vi "质控单元流程.vi"   [LabVIEW 2016]
types:
  T1 = enum16{"步骤1", "步骤2", "步骤3", "步骤4", "步骤5", "步骤6", "步骤7", "步骤8", "步骤9", "步骤10"}
  T2 = enum32{"Bad", "Idle", "Run top level", "Running"}
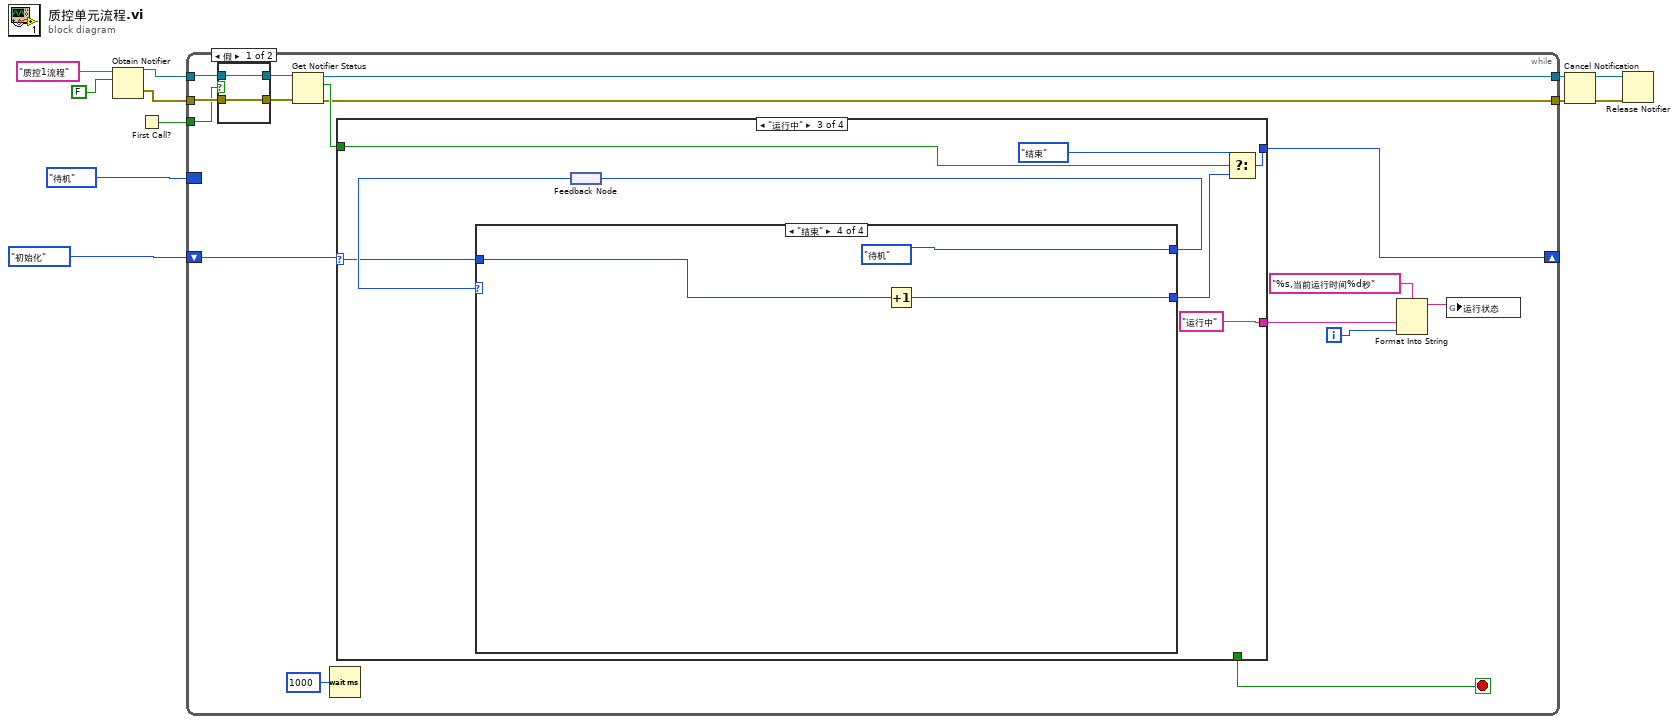
[diagram p0: block diagram]
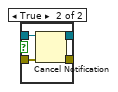
[diagram p2: hidden frame]
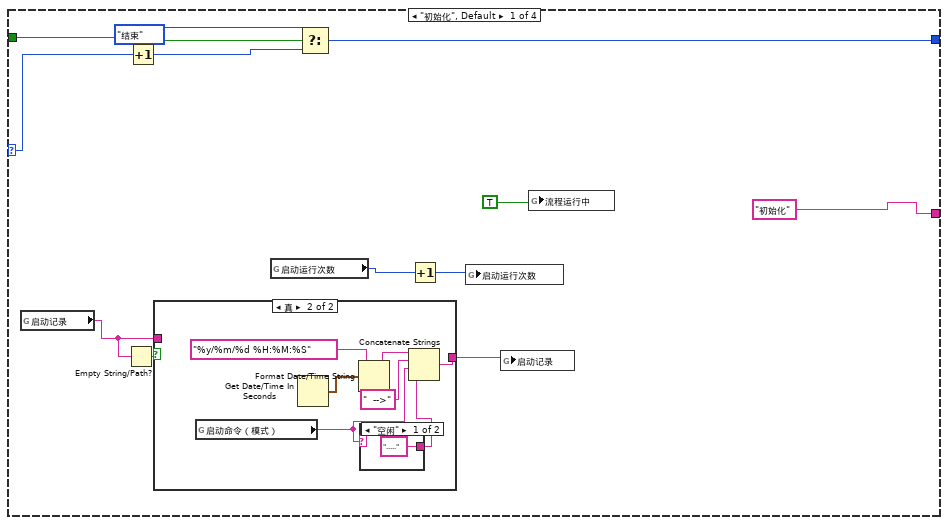
[diagram p3: hidden frame]
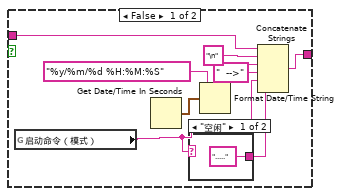
[diagram p4: hidden frame]
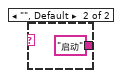
[diagram p5: hidden frame]
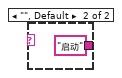
[diagram p6: hidden frame]
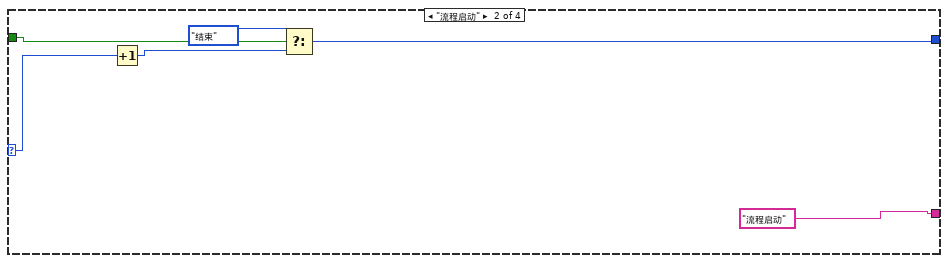
[diagram p7: hidden frame]
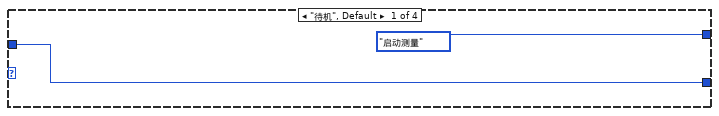
[diagram p8: hidden frame]
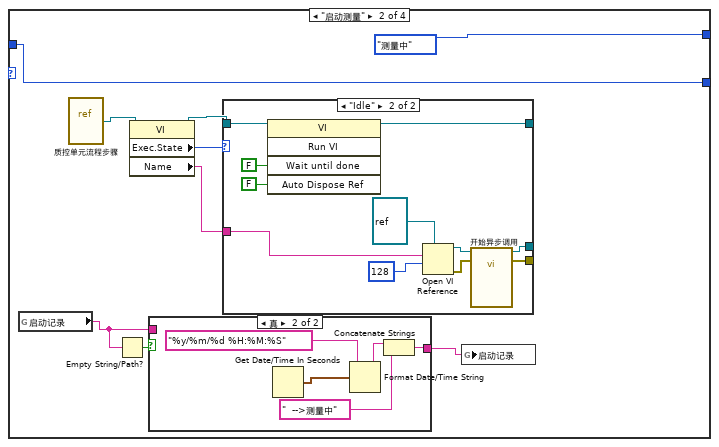
[diagram p9: hidden frame]
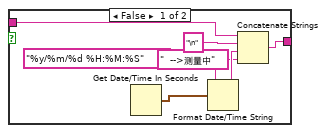
[diagram p10: hidden frame]
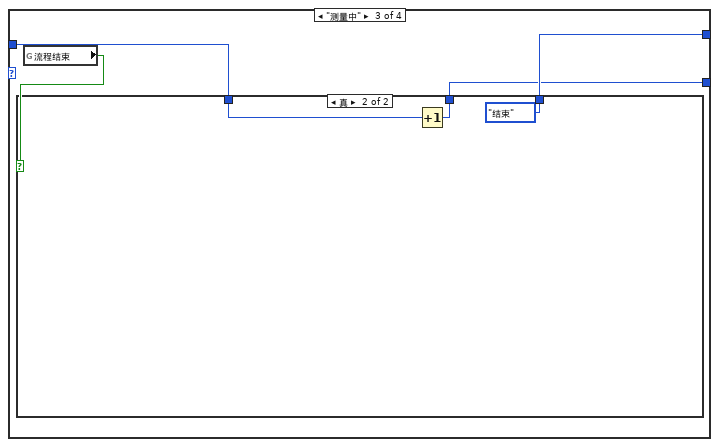
[diagram p12: hidden frame]
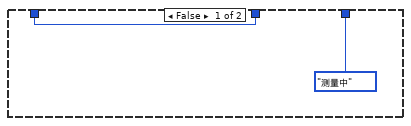
[diagram p13: hidden frame]
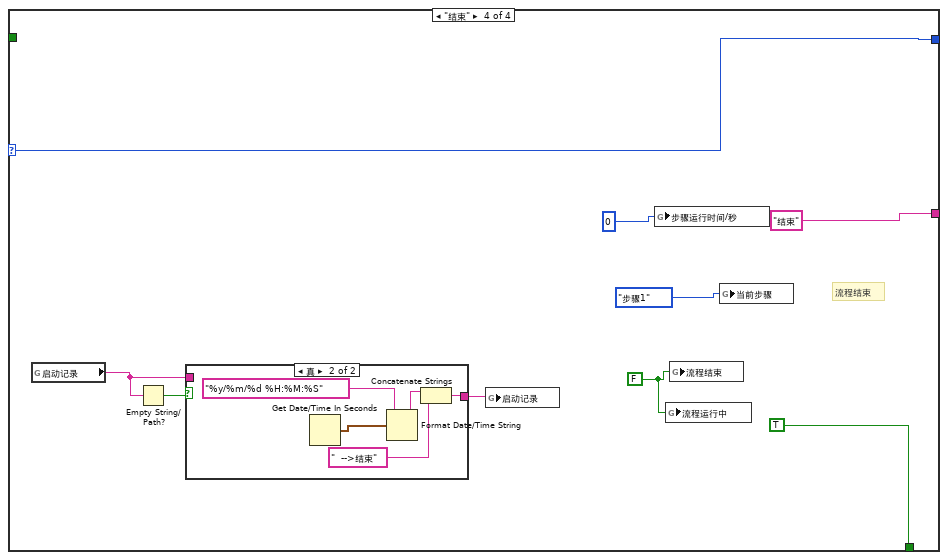
[diagram p14: hidden frame]
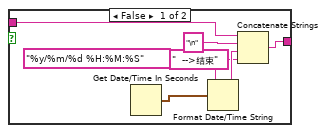
[diagram p15: hidden frame]
diagram:
  n1 = Obtain Notifier(name (unnamed)="质控1流程" ("名称（未命名）"), notification data type=FALSE) -> (notifier out=w8:refnum<notifier>, error out=w7:errorcluster)  [unwired: 2 in, 1 out]
  n2 = First Call?() -> (First Call?: T/F=w1:bool)
  n3 = while {
    shift-right: [w24] -> _
    shift-left: enum16{"初始化", "流程启动", "运行中", "结束"}."初始化" ("枚举") -> [w27]
    tunnel: w8 -> [w16]
    tunnel: w7 -> [w15]
    tunnel: [w19] -> w6
    tunnel: [w18] -> w5
    border: enum16{"待机", "启动测量", "测量中", "结束"}."待机" -> [_]
    tunnel: w1 -> [w12]
    i -> [w22]
    stop <- w20 stop-if-true
    n4 = case shown="假" w12 {
      tunnel: w16 -> [w29 w33]
      tunnel: w15 -> [w28 w32]
      tunnel: [w29 w31] -> w14
      tunnel: [w28 w30] -> w13
      frame False {
      }
      frame True {
        n5 = Cancel Notification(0:w33, 3:w32) -> (8:w31:refnum<notifier>, 11:w30:errorcluster)  [unwired: 1 out]
      }
    }
    n6 = Get Notifier Status(notifier=w14, error in (no error)=w13) -> (notifier out=w19:refnum<notifier>, current notification=w25:bool, error out=w18:errorcluster)  [unwired: 2 out]
    n7 = Wait (ms)(milliseconds to wait=u32 1000 ("等待时间（毫秒）")) -> ()  [unwired: 1 out]
    n8 = case shown="\"运行中\"" w27 {
      selector: w27 -> [w43 w68 w74 w133]
      tunnel: [_ _ _ TRUE ("x")] -> w20
      tunnel: w25 -> [w45 w69 w78 _]
      tunnel: [w41 w67 w73 w133] -> w24
      tunnel: ["初始化" ("输入 1") "流程启动" ("输入 1") "运行中" ("输入 1") "结束" ("输入 1")] -> w21
      frame "初始化", Default {
        n9 = global read "质控单元全局.vi" "启动记录"() -> (w35:string)
        n10 = Empty String/Path?(string/path=w35) -> (empty?=w39:bool)
        n11 = Increment(x=w43) -> (x+1=w42:enum16{"初始化", "流程启动", "运行中", "结束"})
        n12 = case shown="真" w39 {
          tunnel: w35 -> [w54 _]
          tunnel: [w49 w60] -> w34
          frame False {
            n13 = global read "质控单元全局.vi" "启动命令（模式）"() -> (w46:string)
            n14 = Get Date/Time In Seconds() -> (seconds since 1Jan1904=w52:timestamp)
            n15 = case shown="\"空闲\"" w46 {
              tunnel: ["....." ("字符串") "启动" ("字符串")] -> w47
              frame "空闲" {
              }
              frame "", Default {
              }
            }
            n16 = Format Date/Time String(time format string (%c)="%y/%m/%d %H:%M:%S" ("时间格式字符串(%c)"), seconds (now)=w52) -> (date/time string=w50:string)  [unwired: 1 in]
            n17 = Concatenate Strings(w54, "\n" ("字符串"), w50, "  -->" ("字符串"), w46, w47) -> (w49:string)
          }
          frame True {
            n18 = global read "质控单元全局.vi" "启动命令（模式）"() -> (w57:string)
            n19 = Get Date/Time In Seconds() -> (seconds since 1Jan1904=w63:timestamp)
            n20 = Format Date/Time String(time format string (%c)="%y/%m/%d %H:%M:%S" ("时间格式字符串(%c)"), seconds (now)=w63) -> (date/time string=w61:string)  [unwired: 1 in]
            n21 = case shown="\"空闲\"" w57 {
              tunnel: ["....." ("字符串") "启动" ("字符串")] -> w58
              frame "空闲" {
              }
              frame "", Default {
              }
            }
            n22 = Concatenate Strings(w61, "  -->" ("字符串"), w57, w58) -> (w60:string)
          }
        }
        n23 = global read "质控单元全局.vi" "启动运行次数"() -> (w37:i32)
        n24 = Select(t=enum16{"初始化", "流程启动", "运行中", "结束"}."结束" ("枚举"), s=w45, f=w42) -> (s? t:f=w41:enum16{"初始化", "流程启动", "运行中", "结束"})
        n25 = Increment(x=w37) -> (x+1=w36:i32)
        n26 = global write "质控单元全局.vi" "启动运行次数"(w36) -> ()
        n27 = global write "质控单元全局.vi" "启动记录"(w34) -> ()
        n28 = global write "质控单元全局.vi" "流程运行中"(TRUE ("流程运行中")) -> ()
      }
      frame "流程启动" {
        n29 = Increment(x=w68) -> (x+1=w70:enum16{"初始化", "流程启动", "运行中", "结束"})
        n30 = Select(t=enum16{"初始化", "流程启动", "运行中", "结束"}."结束" ("枚举"), s=w69, f=w70) -> (s? t:f=w67:enum16{"初始化", "流程启动", "运行中", "结束"})
      }
      frame "运行中" {
        n31 = feedback #1() -> (w77:enum16{"待机", "启动测量", "测量中", "结束"})
        n32 = case shown="\"结束\"" w77 {
          tunnel: [enum16{"待机", "启动测量", "测量中", "结束"}."启动测量" enum16{"待机", "启动测量", "测量中", "结束"}."测量中" w118 enum16{"待机", "启动测量", "测量中", "结束"}."待机"] -> w76
          tunnel: [w80 w89 w116 w125] -> w75
          tunnel: w74 -> [w80 w89 w117 w124]
          frame "待机", Default {
          }
          frame "启动测量" {
            n33 = global read "质控单元全局.vi" "启动记录"() -> (w83:string)
            n34 = vi-ref "质控单元流程步骤.vi"() -> (w85:refnum<vi>)
            n35 = Empty String/Path?(string/path=w83) -> (empty?=w84:bool)
            n36 = property class="VI"(reference=w85) -> (reference out=w86:refnum<vi>, "Exec.State"=w87:T2, "Name"=w88:string)  [unwired: 1 in, 1 out]
            n37 = case shown="真" w84 {
              tunnel: w83 -> [w97 _]
              tunnel: [w91 w98] -> w82
              frame False {
                n38 = Get Date/Time In Seconds() -> (seconds since 1Jan1904=w95:timestamp)
                n39 = Format Date/Time String(time format string (%c)="%y/%m/%d %H:%M:%S" ("时间格式字符串(%c)"), seconds (now)=w95) -> (date/time string=w93:string)  [unwired: 1 in]
                n40 = Concatenate Strings(w97, "\n" ("字符串"), w93, "  -->测量中" ("字符串")) -> (w91:string)
              }
              frame True {
                n41 = Get Date/Time In Seconds() -> (seconds since 1Jan1904=w102:timestamp)
                n42 = Format Date/Time String(time format string (%c)="%y/%m/%d %H:%M:%S" ("时间格式字符串(%c)"), seconds (now)=w102) -> (date/time string=w100:string)  [unwired: 1 in]
                n43 = Concatenate Strings(w100, "  -->测量中" ("字符串")) -> (w98:string)
              }
            }
            n44 = case shown="\"Idle\"" w87 {
              tunnel: w86 -> [w103 w111]
              tunnel: [w103 w112] -> _
              tunnel: w88 -> [_ w110]
              tunnel: [_ w105] -> _
              tunnel: [_ w104] -> _
              frame "Bad", Default {
              }
              frame "Idle" {
                n45 = invoke class="VI" method="Run VI"(reference=w111, "Wait until done"=FALSE ("结束前等待"), "Auto Dispose Ref"=FALSE ("自动销毁引用")) -> (reference out=w112:refnum<vi>)  [unwired: 2 in, 4 out]
                n46 = Open VI Reference(type specifier VI Refnum (for type only)=refnum<vi> refnum ("类型说明符VI引用句柄（仅用于类型）"), vi path=w110, options=128 ("选项")) -> (vi reference=w106:refnum<vi>, error out=w108:errorcluster)  [unwired: 3 in]
                n47 = call-by-ref "开始异步调用"(reference=w106, error in=w108) -> (reference out=w105:refnum<vi>, error out=w104:errorcluster)  [unwired: 12 in]
              }
            }
            n48 = global write "质控单元全局.vi" "启动记录"(w82) -> ()
          }
          frame "测量中" {
            n49 = global read "质控单元全局.vi" "流程结束"() -> (w115:bool)
            n50 = case shown="真" w115 {
              tunnel: [enum16{"待机", "启动测量", "测量中", "结束"}."测量中" enum16{"待机", "启动测量", "测量中", "结束"}."结束"] -> w118
              tunnel: w117 -> [w119 w122]
              tunnel: [w119 w121] -> w116
              frame False {
              }
              frame True {
                n51 = Increment(x=w122) -> (x+1=w121:enum16{"初始化", "流程启动", "运行中", "结束"})
              }
            }
          }
          frame "结束" {
            n52 = Increment(x=w124) -> (x+1=w125:enum16{"初始化", "流程启动", "运行中", "结束"})
          }
        }
        n53 = feedback-in #1(w76) -> ()
        n54 = Select(t=enum16{"初始化", "流程启动", "运行中", "结束"}."结束" ("枚举"), s=w78, f=w75) -> (s? t:f=w73:enum16{"初始化", "流程启动", "运行中", "结束"})
      }
      frame "结束" {
        w131 = FALSE ("流程结束")
        # "流程结束"
        n55 = global read "质控单元全局.vi" "启动记录"() -> (w127:string)
        n56 = Empty String/Path?(string/path=w127) -> (empty?=w132:bool)
        n57 = case shown="真" w132 {
          tunnel: w127 -> [w142 _]
          tunnel: [w136 w143] -> w128
          frame False {
            n58 = Get Date/Time In Seconds() -> (seconds since 1Jan1904=w140:timestamp)
            n59 = Format Date/Time String(time format string (%c)="%y/%m/%d %H:%M:%S" ("时间格式字符串(%c)"), seconds (now)=w140) -> (date/time string=w138:string)  [unwired: 1 in]
            n60 = Concatenate Strings(w142, "\n" ("字符串"), w138, "  -->结束" ("字符串")) -> (w136:string)
          }
          frame True {
            n61 = Get Date/Time In Seconds() -> (seconds since 1Jan1904=w147:timestamp)
            n62 = Format Date/Time String(time format string (%c)="%y/%m/%d %H:%M:%S" ("时间格式字符串(%c)"), seconds (now)=w147) -> (date/time string=w145:string)  [unwired: 1 in]
            n63 = Concatenate Strings(w145, "  -->结束" ("字符串")) -> (w143:string)
          }
        }
        n64 = global write "质控单元全局.vi" "启动记录"(w128) -> ()
        n65 = global write "质控单元全局.vi" "步骤运行时间/秒"(0 ("运行时间/秒")) -> ()
        n66 = global write "质控单元全局.vi" "流程运行中"(w131) -> ()
        n67 = global write "质控单元全局.vi" "流程结束"(w131) -> ()
        n68 = global write "质控单元全局.vi" "当前步骤"(T1."步骤1" ("当前步骤 2")) -> ()
      }
    }
    n69 = Format Into String(format string="%s,当前运行时间%d秒" ("格式字符串"), w21, w22) -> (resulting string=w17:string)  [unwired: 2 in, 1 out]
    n70 = global write "质控单元全局.vi" "运行状态"(w17) -> ()
  }
  n71 = Cancel Notification(0:w6, 3:w5) -> (8:w4:refnum<notifier>, 11:w3:errorcluster)  [unwired: 1 out]
  n72 = Release Notifier(notifier=w4, error in (no error)=w3) -> ()  [unwired: 1 in, 3 out]
